vi "Get Build Specification Version.vi"   [LabVIEW 2020, in "NI_App_Builder_API.lvlib"]
doc: "Gets the version information of a build specification. This VI returns the <B>Major, Minor, Fix</B>, and <B>Build</B> version numbers, which correspond to the version numbers on the <B>Version Information</B> page of the properties dialog box for the build specification."
uses:
  <vilib>/AppBuilder/AB_API_Simple/NI_App_Builder_API.lvlib
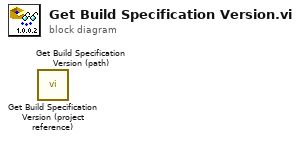
[diagram p0: block diagram]
diagram:
  n1 = call <vilib>:"Get Build Specification Version (project reference).vi"() -> ()  [unwired: 9 in, 3 out]
  n2 = call <vilib>:"Get Build Specification Version (path).vi"() -> ()  [unwired: 10 in, 2 out]
